vi "HGF_TaskOnce.appendData2Variant.vi"(0 "initData":variant, 5 "error in (no error)":errorcluster) -> (14 "dup initData":variant, 19 "error out":errorcluster)   [LabVIEW 2014, in "HGF_BaseClasses.lvlib" / "HGF_TaskOnce.lvclass"]
doc: "Append initialize data to variant."
uses:
  HGF_TaskOnce.lvclass
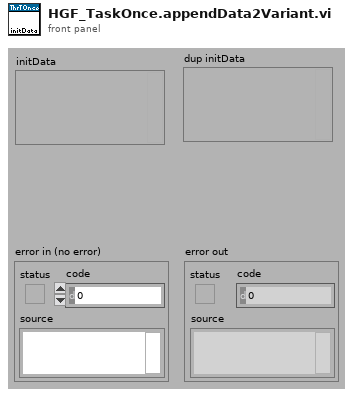
[diagram p1: front panel]
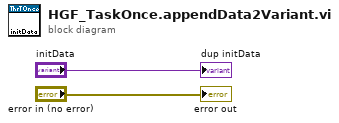
[diagram p0: block diagram]
diagram:
  "dup initData" <- "initData"
  "error out" <- "error in (no error)"
